vi "gradient_descent.vi"(8 "alpha":dbl, 9 "iterations":i32, 10 "Y in":dbl[](array[numeric]), 11 "X in":dbl[][](array[numeric])) -> (0 "W2":dbl[][](array[numeric]), 1 "b1":dbl[](array[numeric]), 2 "accuracy":dbl[](array[numeric]), 3 "W1":dbl[][](array[numeric]), 4 "b2":dbl[](array[numeric]), 5 "X out":dbl[][](array[numeric]), 6 "predictions":dbl[][](array[numeric]), 7 "Y out":dbl[](array[numeric]))   [LabVIEW 2023]
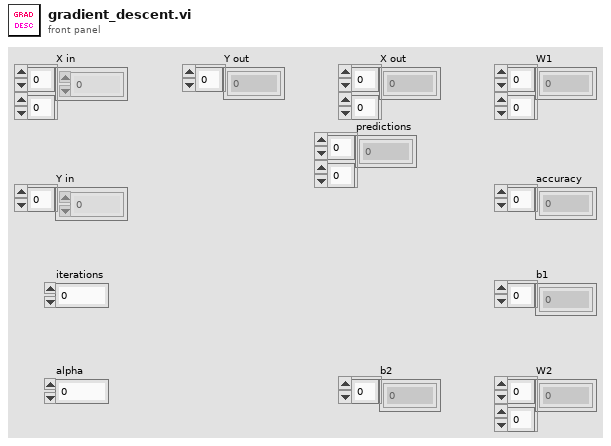
[diagram p1: front panel]
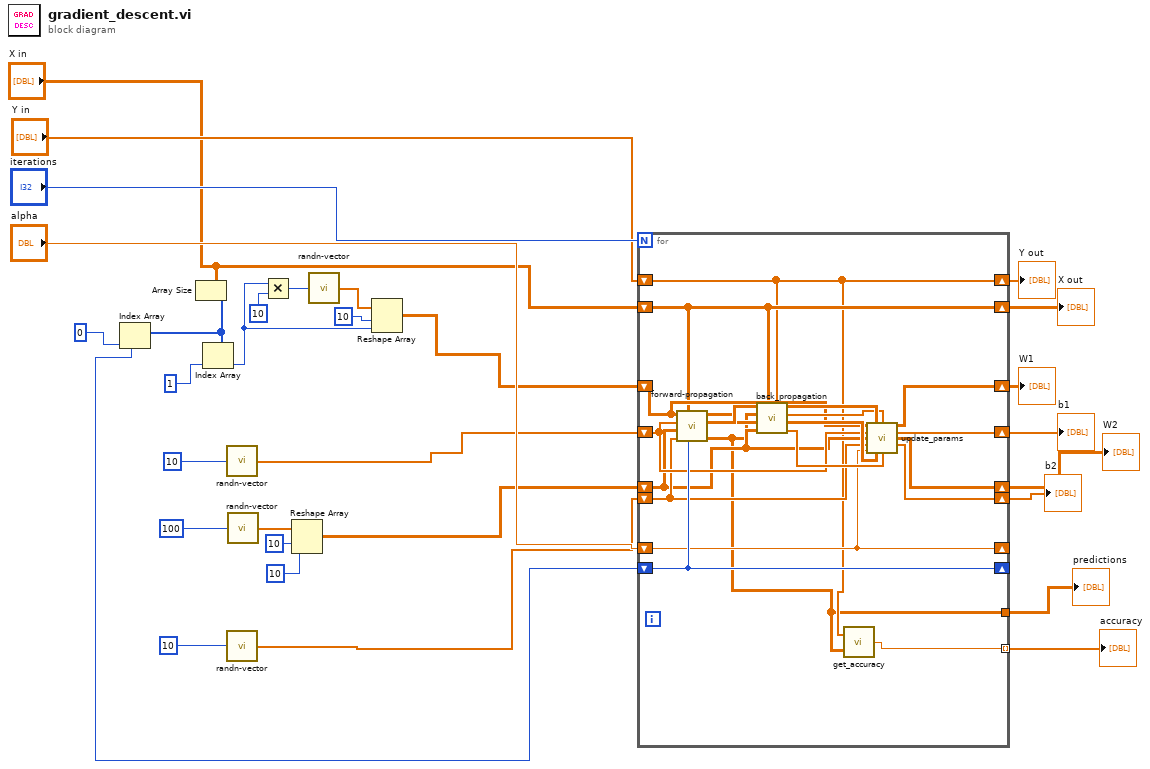
[diagram p0: block diagram]
diagram:
  n1 = Array Size(array="X in") -> (size(s)=w8:i32[])
  n2 = Index Array(array=w8, index=0) -> (element=w21:i32)
  n3 = Index Array(array=w8, index=1) -> (element=w5:i32)
  n4 = call "randn-vector.vi"("Numeric"=10) -> ("Array"=w18:dbl[])
  n5 = call "randn-vector.vi"("Numeric"=10) -> ("Array"=w20:dbl[])
  n6 = call "randn-vector.vi"("Numeric"=100) -> ("Array"=w14:dbl[])
  n7 = Multiply(x=w5, y=10) -> (x*y=w10:i32)
  n8 = Reshape Array(w14, 10 ("dimension size"), 10 ("dimension size")) -> (w19:dbl[][])
  n9 = call "randn-vector.vi"("Numeric"=w10) -> ("Array"=w11:dbl[])
  n10 = Reshape Array(w11, 10 ("dimension size"), w5) -> (w17:dbl[][])
  n11 = for {
    N: "iterations" -> [_]
    shift-right: [w38] -> w27
    shift-left: w19 -> [w35]
    shift-right: [w39] -> w26
    shift-left: w18 -> [w44]
    shift-right: [w40] -> w25
    shift-left: w17 -> [w45]
    shift-right: [w41] -> w31
    shift-left: "X in" -> [w41]
    shift-right: [w37] -> w28
    shift-left: w20 -> [w43]
    shift-right: [w46] -> _
    shift-left: w21 -> [w46]
    shift-right: [w34] -> w30
    shift-left: "Y in" -> [w34]
    shift-right: [w42] -> _
    shift-left: "alpha" -> [w42]
    tunnel: [w33] -> w29 mode=indexing
    tunnel: [w32] -> w1
    n12 = call "forward-propagation.vi"("Number of Examples"=w46, "X"=w41, "b2"=w43, "W2"=w35, "b1"=w44, "W1"=w45) -> ("A2"=w32:dbl[][], "A1"=w51:dbl[][], "Z1"=w36:dbl[][])  [unwired: 2 in, 1 out]
    n13 = call "back_propagation.vi"("Y"=w34, "X"=w41, "W2"=w35, "Z1"=w36, "A2"=w32, "A1"=w51) -> ("db2"=w47:dbl[], "dW2"=w48:dbl[][], "db1"=w49:dbl[], "dW1"=w50:dbl[][])  [unwired: 2 in]
    n14 = call "get_accuracy.vi"("predict"=w32, "Y"=w34) -> ("accuracy"=w33:dbl)
    n15 = call "update_params.vi"("W1 in"=w45, "dW1"=w50, "db1"=w49, "b1 in"=w44, "W2 in"=w35, "b2 in"=w43, "alpha"=w42, "dW2"=w48, "db2"=w47) -> ("W1 out"=w40:dbl[][], "b1 out"=w39:dbl[], "W2 out"=w38:dbl[][], "b2 out"=w37:dbl[])  [unwired: 3 in]
  }
  "W1" <- w25
  "b1" <- w26
  "W2" <- w27
  "b2" <- w28
  "accuracy" <- w29
  "Y out" <- w30
  "X out" <- w31
  "predictions" <- w1
